vi "calibrate_temp.vi"(1 "in":dbl) -> (0 "out":dbl)   [LabVIEW 2023]
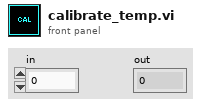
[diagram p1: front panel]
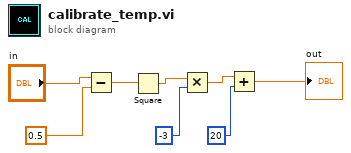
[diagram p0: block diagram]
diagram:
  n1 = Subtract(x="in", y=0.5) -> (x-y=w6:dbl)
  n2 = Square(x=w6) -> (x^2=w5:dbl)
  n3 = Multiply(x=w5, y=-3) -> (x*y=w3:dbl)
  n4 = Add(x=w3, y=20) -> (x+y=→"out":dbl)
